vi "Render Copy (Destination Rect As Cluster).vi"(6 "Destination Rectangle":T1, 9 "Source Rectangle Pointer":u32 format="%.0x", 10 "Texture Pointer":u32 format="%.0x", 11 "Renderer Pointer":u32 format="%.0x") -> (3 "Return":i32)   [LabVIEW 2015, in "LibSDL2.lvlib"]
uses:
  LibSDL2.lvlib
  Controls/Rectangle.ctl
  DLL/SDL2.dll
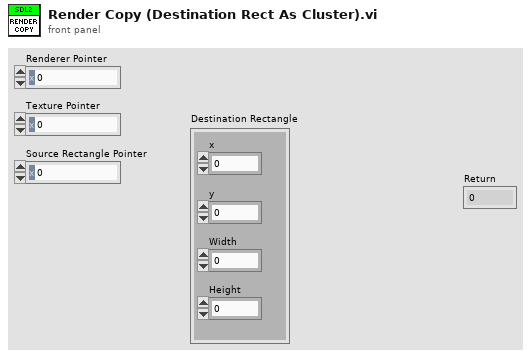
[diagram p1: front panel]
types:
  T1 = typedef "LibSDL2.lvlib/Rectangle.ctl" = cluster{"x":i32, "y":i32, "Width":i32, "Height":i32}
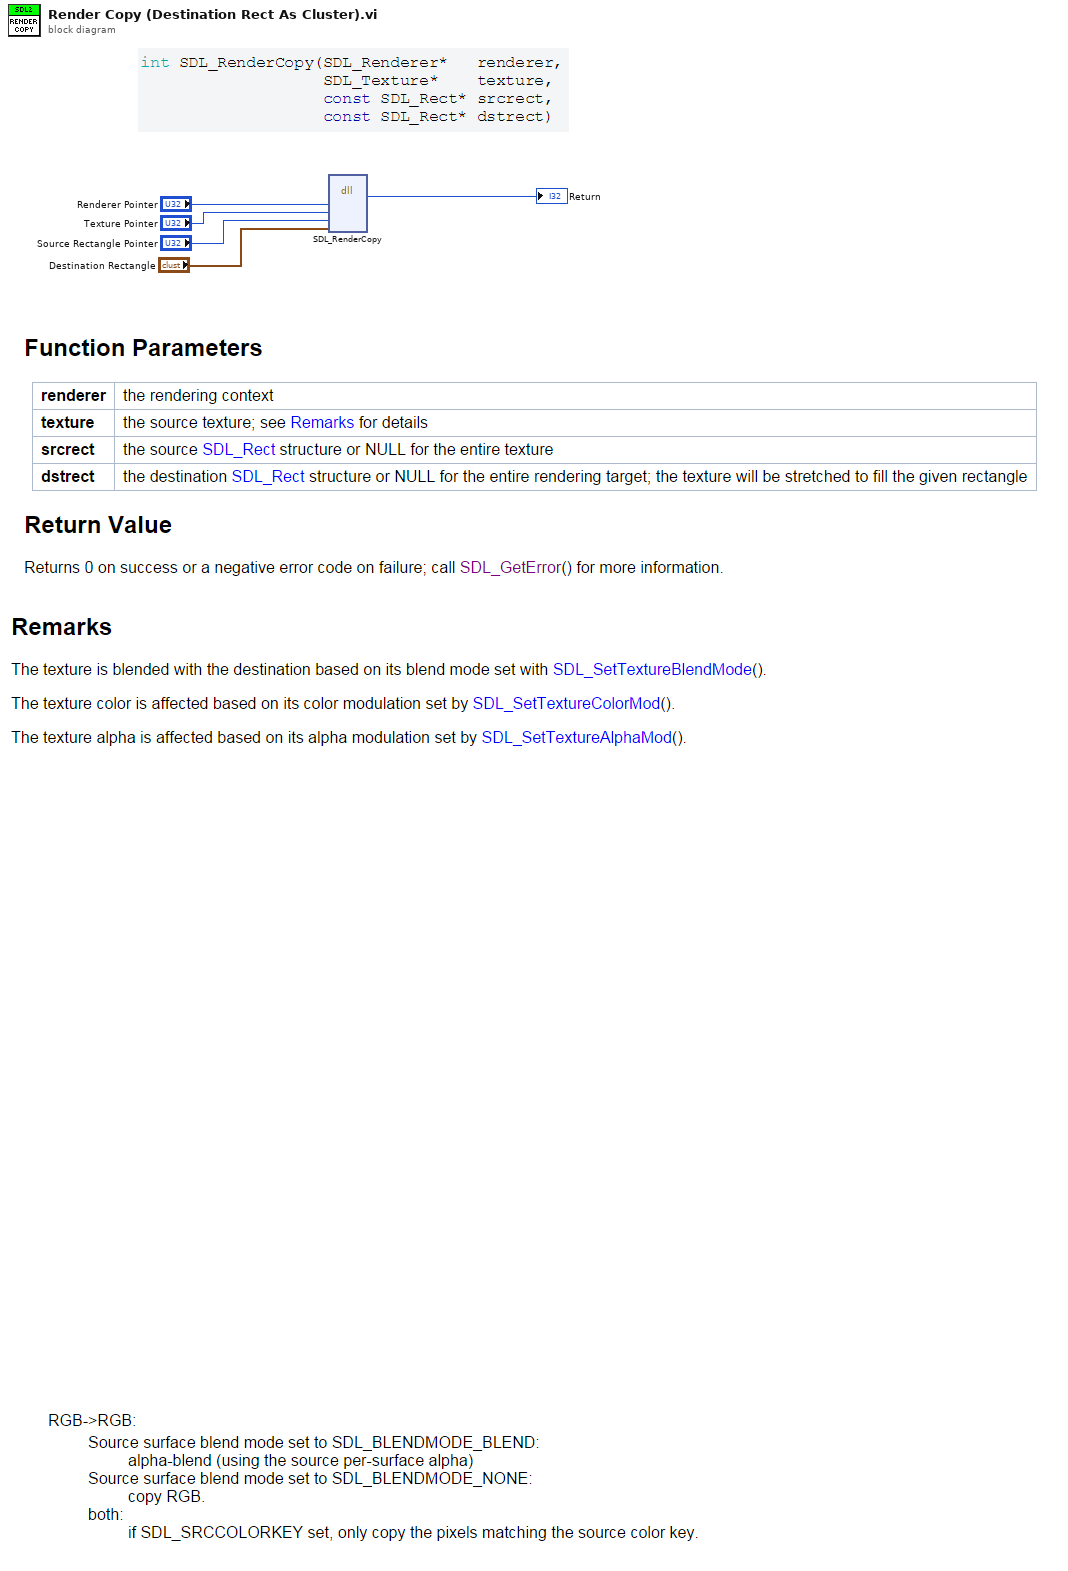
[diagram p0: block diagram]
diagram:
  n1 = dll-call lib="C:/dev/PGS/LabSDL2/Source/Libraries/LibSDL2 Wrapper/DLL/SDL2.dll" fn="SDL_RenderCopy"("renderer_pointer"="Renderer Pointer", "texture_pointer"="Texture Pointer", "srcrect_pointer"="Source Rectangle Pointer", "dstrect_pointer"="Destination Rectangle") -> ("return type"=→"Return":i32)  [unwired: 7 in, 2 out]
